vi "engine.vi"(8 "error in":errorcluster, 10 "clk (NaN)":dbl=nan, 11 "Procedure in":variant[](array[variant])=[variant("procCLK"=variant(dbl 3802946268.2064614), "procIndex"=variant(dbl 2.0), "procIsRunning"=variant(bool TRUE), "procLabel"=variant(string "blink-2"), "procRegisterNumeric"=variant(dbl 3802946266.867457), "procReport"=variant(string "blink-2:3802946268,2>>2,_DELAY_COMPARE,1.3/2.0,STAY"), "procReportPast"=variant(string "blink-2:3802946268,2>>2,_DELAY_COMPARE,1.3/2.0,STAY")), variant("stepFunction"=variant(enum16{"__NO-OP", "_DELAY_LOAD", "_DELAY_COMPARE", "_COMPARE", "_JUMP", "_FINISH", "CLK_COMPARE", "PROC_START", "PROC_STOP", "PROC_ISRUN_COMPARE", "PROC_ISRUN_LOAD", "_IO_READ_IN", "_IO_WRITE_DOUT", "_IO_COMPARE", "Q_OPEN", "Q_WRITE", "Q_READ"} enum."_IO_WRITE_DOUT"), "stepIoPointer"=variant(string "dout2"), "stepIoState(str)"=variant(string "1:1"), "stepLabel"=variant(string "loop"), "stepPath"=variant(string "")), variant("stepFunction"=variant(enum16{"__NO-OP", "_DELAY_LOAD", "_DELAY_COMPARE", "_COMPARE", "_JUMP", "_FINISH", "CLK_COMPARE", "PROC_START", "PROC_STOP", "PROC_ISRUN_COMPARE", "PROC_ISRUN_LOAD", "_IO_READ_IN", "_IO_WRITE_DOUT", "_IO_COMPARE", "Q_OPEN", "Q_WRITE", "Q_READ"} enum."_DELAY_LOAD"), "stepLabel"=variant(string "")), variant("stepFunction"=variant(enum16{"__NO-OP", "_DELAY_LOAD", "_DELAY_COMPARE", "_COMPARE", "_JUMP", "_FINISH", "CLK_COMPARE", "PROC_START", "PROC_STOP", "PROC_ISRUN_COMPARE", "PROC_ISRUN_LOAD", "_IO_READ_IN", "_IO_WRITE_DOUT", "_IO_COMPARE", "Q_OPEN", "Q_WRITE", "Q_READ"} enum."_DELAY_COMPARE"), "stepSetpoint"=variant(cluster{"comparison":string, "Y":dbl} {"comparison"="", "Y"=2.0})), variant("stepFunction"=variant(enum16{"__NO-OP", "_DELAY_LOAD", "_DELAY_COMPARE", "_COMPARE", "_JUMP", "_FINISH", "CLK_COMPARE", "PROC_START", "PROC_STOP", "PROC_ISRUN_COMPARE", "PROC_ISRUN_LOAD", "_IO_READ_IN", "_IO_WRITE_DOUT", "_IO_COMPARE", "Q_OPEN", "Q_WRITE", "Q_READ"} enum."_JUMP"), "stepLabel"=variant(string ""), "stepPointer"=variant(string "loop"))]) -> (0 "error out":errorcluster, 1 "cmdEng":cluster{"CMD":T2, "data":variant}={"CMD"=enum."ENG.PROC.ISRUNNING", "data"=variant}, 2 "Q-Log Command":cluster{"data":variant, "Enum":T1}={"data"=variant, "Enum"=enum."LOG.CATCH"}, 3 "Procedure out":variant[](array[variant])=[variant("procCLK"=variant(dbl 3802946268.216451), "procIndex"=variant(dbl 2.0), "procIsRunning"=variant(bool TRUE), "procLabel"=variant(string "blink-2"), "procRegisterNumeric"=variant(dbl 3802946266.867457), "procReport"=variant(string "blink-2:3802946268,2>>2,_DELAY_COMPARE,1.3/2.0,STAY"), "procReportPast"=variant(string "blink-2:3802946268,2>>2,_DELAY_COMPARE,1.3/2.0,STAY")), variant("stepFunction"=variant(enum16{"__NO-OP", "_DELAY_LOAD", "_DELAY_COMPARE", "_COMPARE", "_JUMP", "_FINISH", "CLK_COMPARE", "PROC_START", "PROC_STOP", "PROC_ISRUN_COMPARE", "PROC_ISRUN_LOAD", "_IO_READ_IN", "_IO_WRITE_DOUT", "_IO_COMPARE", "Q_OPEN", "Q_WRITE", "Q_READ"} enum."_IO_WRITE_DOUT"), "stepIoPointer"=variant(string "dout2"), "stepIoState(str)"=variant(string "1:1"), "stepLabel"=variant(string "loop"), "stepPath"=variant(string "")), variant("stepFunction"=variant(enum16{"__NO-OP", "_DELAY_LOAD", "_DELAY_COMPARE", "_COMPARE", "_JUMP", "_FINISH", "CLK_COMPARE", "PROC_START", "PROC_STOP", "PROC_ISRUN_COMPARE", "PROC_ISRUN_LOAD", "_IO_READ_IN", "_IO_WRITE_DOUT", "_IO_COMPARE", "Q_OPEN", "Q_WRITE", "Q_READ"} enum."_DELAY_LOAD"), "stepLabel"=variant(string "")), variant("stepFunction"=variant(enum16{"__NO-OP", "_DELAY_LOAD", "_DELAY_COMPARE", "_COMPARE", "_JUMP", "_FINISH", "CLK_COMPARE", "PROC_START", "PROC_STOP", "PROC_ISRUN_COMPARE", "PROC_ISRUN_LOAD", "_IO_READ_IN", "_IO_WRITE_DOUT", "_IO_COMPARE", "Q_OPEN", "Q_WRITE", "Q_READ"} enum."_DELAY_COMPARE"), "stepSetpoint"=variant(cluster{"comparison":string, "Y":dbl} {"comparison"="", "Y"=2.0})), variant("stepFunction"=variant(enum16{"__NO-OP", "_DELAY_LOAD", "_DELAY_COMPARE", "_COMPARE", "_JUMP", "_FINISH", "CLK_COMPARE", "PROC_START", "PROC_STOP", "PROC_ISRUN_COMPARE", "PROC_ISRUN_LOAD", "_IO_READ_IN", "_IO_WRITE_DOUT", "_IO_COMPARE", "Q_OPEN", "Q_WRITE", "Q_READ"} enum."_JUMP"), "stepLabel"=variant(string ""), "stepPointer"=variant(string "loop"))], 4 "Continue?":bool)   [LabVIEW 2024]
uses:
  controls/state-engine.ctl
  controls/state-logger.ctl
  controls/type.eng.log-cluster.ctl
  controls/typeCmdPostStepFunc.ctl
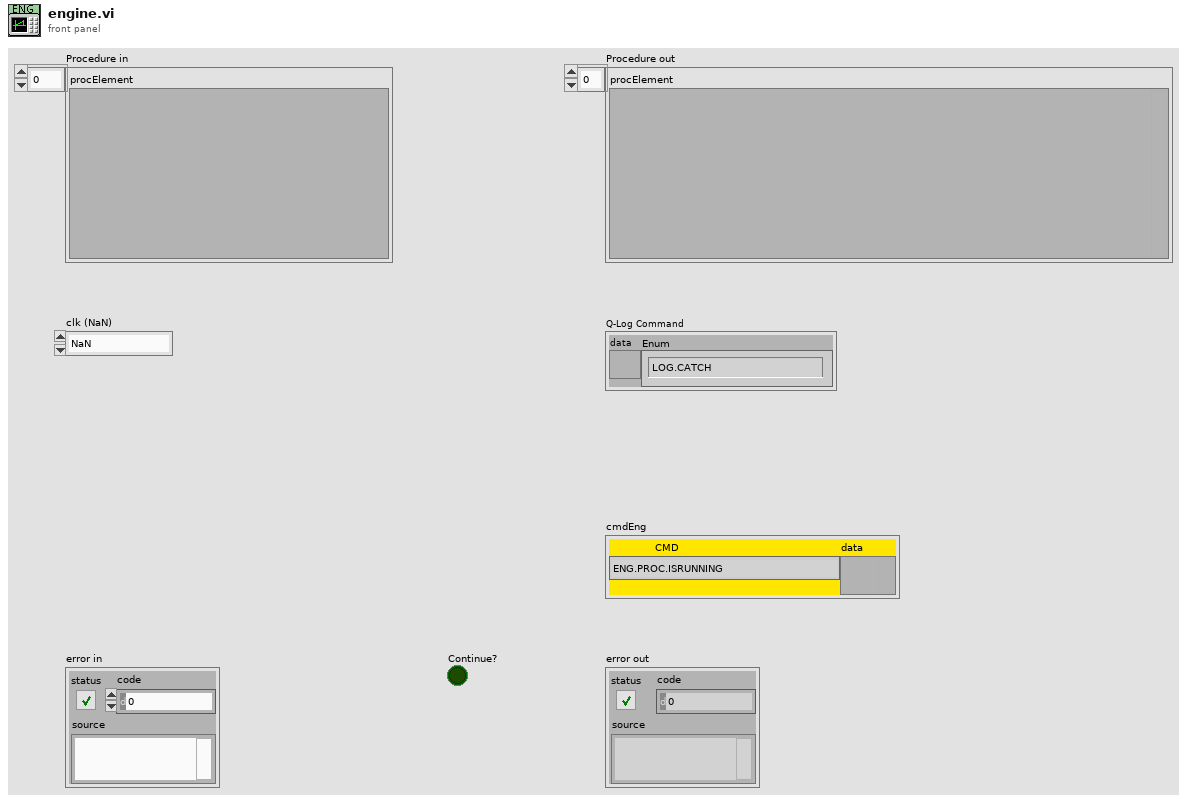
[diagram p1: front panel]
types:
  T1 = typedef "state-logger.ctl" = enum16{"LOG.NO_OP", "LOG.INIT", "LOG.INIT.NTR-FLOW", "LOG.EXIT", "LOG.CATCH", "LOG.PARSE.OCS", "LOG.UPDATE.SELECTORS", "LOG.UPDATE.IRR", "LOG.SNAPSHOT.PROC", "LOG.SNAPSHOT"}
  T2 = typedef "state-engine.ctl" = enum16{"ENG.NO-OP", "ENG.START", "ENG.STOP", "ENG.EXECUTE", "ENG.STATUS", "ENG.EXTERNAL-CALL", "ENG.INIT", "ENG.INIT.VARS", "ENG.INIT.SERIAL", "ENG.LOAD", "ENG.LOAD.SINGLE", "ENG.LOAD.MODULE", "ENG.LOAD.RELOAD", "ENG.LOAD.UNLOAD", "ENG.IO.LOAD", "ENG.IO.SAVE", "ENG.PROC.RELOAD-BY-NAME", "ENG.PROC.START", "ENG.PROC.STOP", "ENG.PROC.INSERT-STEPS", "ENG.PROC.ISRUNNING", "ENG.PROC.PRESET", "ENG.PROC.STATUS", "ENG.PRINT-USER-MSG", "ENG.RIO.SNAPSHOT", "ENG.RIO.AIN-SNAPSHOT-CALIB", "ENG.RIO.DOUT-BY-ADDR", "ENG.RIO.DOUT-BY-NAME", "ENG.RIO.RFS-DELAY-SET-X1", "ENG.RIO.RFS-DELAY-SET-X8", "ENG.RIO.RFS-CYCLES-SET", "ENG.RIO.RFS-CYCLES-GET", "ENG.RIO.RFS-ENABLE", "ENG.EXIT"}
  T3 = typedef "type.eng.log-cluster.ctl" = cluster{"Procedure(post)":variant[], "Procedure(pre)":variant[], "Next State ":cluster{"CMD":T4, "data":variant}, "IsRunning":bool, "error in":errorcluster}
  T4 = typedef "typeCmdPostStepFunc.ctl" = enum16{"NEXT", "PREV", "JUMP", "STAY", "COMPLETE", "ENGCALL.PROC.START", "ENGCALL.PROC.STOP", "ENGCALL.PROC.COMPLETION-CHECK", "ENGCALL.PROC.INIT", "ERROR"}
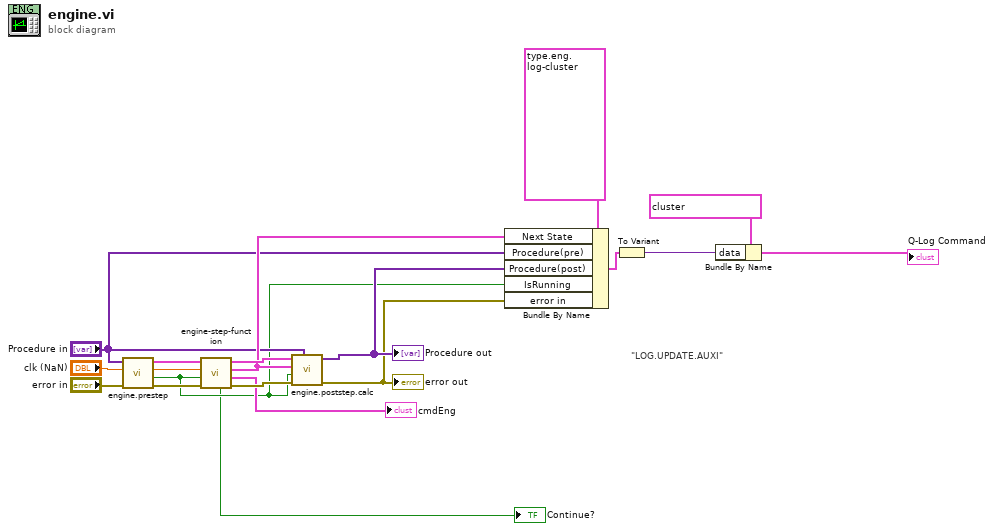
[diagram p0: block diagram]
diagram:
  # "\"LOG.UPDATE.AUXI\""
  n1 = call "engine.prestep.vi"("error in"="error in", "clk(NaN)"="clk (NaN)", "proc in"="Procedure in") -> ("error out"=w17:errorcluster, "isRunning"=w4:bool, "sysClk out"=w16:dbl, "HeaderElement out"=w18:cluster{variant[]})  [unwired: 5 in]
  n2 = call "engine-step-function.vi"("error in (no error)"=w17, "isRunning?"=w4, "clk"=w16, "HeaderElement in"=w18) -> ("error out"=w14:errorcluster, "ENG.CALL"=→"cmdEng":cluster{"CMD":T2, "data":variant}, "Next State in"=w10:cluster{"CMD":T4, "data":variant}, "HeaderElement out"=w15:cluster{variant[]}, "continue?"=→"Continue?":bool)  [unwired: 3 in]
  n3 = call "engine.poststep.calc.vi"("Procedure(pre)"="Procedure in", "error in"=w14, "isRunning?(T)"=w4, "Next State in"=w10, "HeaderElement in"=w15) -> ("error out"=w3:errorcluster, "Procedure Out"=w8:variant[])  [unwired: 5 in]
  "Procedure out" <- w8
  "error out" <- w3
  n4 = Bundle By Name(cluster=T3 {"Procedure(post)"=[], "Procedure(pre)"=[], "Next State "={"CMD"=enum."NEXT", "data"=variant}, "IsRunning"=FALSE, "error in"={"status"=FALSE, "code"=0, "source"=""}}, "Next State"=w10, "Procedure(pre)"="Procedure in", "Procedure(post)"=w8, "IsRunning"=w4, "error in"=w3) -> (w7:T3)
  n5 = To Variant(anything=w7) -> (Variant=w5:variant)
  n6 = Bundle By Name(cluster=cluster{"data":variant, "Enum":T1} {"data"=variant, "Enum"=enum."LOG.CATCH"} ("procQ"), "data"=w5) -> (→"Q-Log Command":cluster{"data":variant, "Enum":T1})
